vi "RetrieveMetadataLiveOrPost.vi"(11 "Array in":string[](array[string])) -> (3 "Array out":dbl[](array[numeric]))   [LabVIEW 2015]
doc: "Given the Time Data Was Acquired (from MeasGlobal) in Take New Data mode, or Raw Data file (from MeasGlobal) in Post Process mode, this VI retrieves single values of the requested ADAM channels for the current measurement."
uses:
  Anemometry/Anemometry Sub Vis/Globals/Meas_global.vi
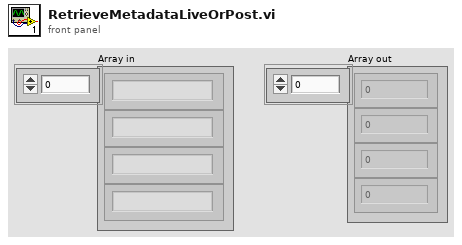
[diagram p1: front panel]
types:
  T1 = typedef "Post_Process.ctl" = enum16{"Take New Data", "Post Process Raw Data File"}
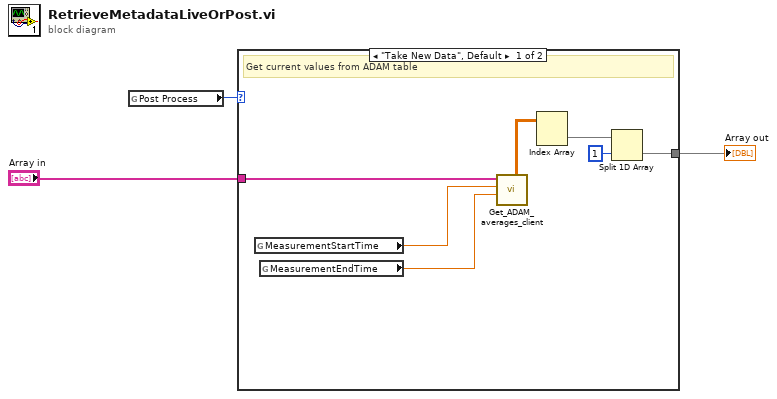
[diagram p0: block diagram]
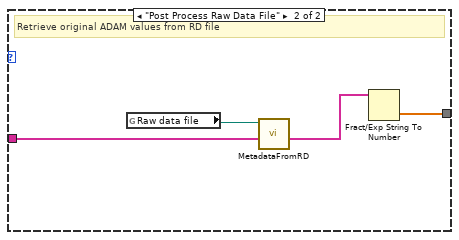
[diagram p2: hidden frame]
diagram:
  n1 = global read "Meas_global.vi" "Post Process"() -> (w2:T1)
  n2 = case shown="\"Take New Data\", Default" w2 {
    tunnel: "Array in" -> [w10 w13]
    tunnel: [w6 w11] -> w3
    frame "Take New Data", Default {
      # "Get current values from ADAM table"
      n3 = global read "Meas_global.vi" "MeasurementStartTime"() -> (w5:dbl)
      n4 = global read "Meas_global.vi" "MeasurementEndTime"() -> (w4:dbl)
      n5 = call "Get_ADAM_averages_client.vi"("End time"=w4, "Start time"=w5, "ADAM Ch Names"=w10) -> ("DBL values"=w9:dbl[][])  [unwired: 4 in, 4 out]
      n6 = Index Array(array=w9) -> (element=w8:dbl[])  [unwired: 2 in]
      n7 = Split 1D Array(array=w8, index=1) -> (second subarray=w6:dbl[])  [unwired: 1 out]
    }
    frame "Post Process Raw Data File" {
      (unwired) string[] []
      # "Retrieve original ADAM values from RD file"
      n8 = global read "Meas_global.vi" "Raw data file"() -> (w14:path)
      n9 = call "MetadataFromRD.vi"("ChannelNames"=w13, "Raw data file"=w14) -> ("ValueStrings"=w12:string[])  [unwired: 8 in, 1 out]
      n10 = Fract/Exp String To Number(string=w12) -> (number=w11:dbl[])  [unwired: 3 in, 1 out]
    }
  }
  "Array out" <- w3
